vi "OSC UDP Receiver.vi"() -> ()   [LabVIEW 2013]
doc: "This example VI shows how to read Open Sound Control (OSC) messages from UDP and dispatch them by their OSC address patterns. This VI is intended to be run with the OSC UDP Sender example VI."
uses:
  <vilib>/NIOSC/Argument to Float32 Data.vi
  <vilib>/NIOSC/Argument to Boolean Data.vi
  <vilib>/NIOSC/Argument to String Data.vi
  <vilib>/NIOSC/Argument to Double Data.vi
  <vilib>/NIOSC/Generate Error.vi
  <vilib>/NIOSC/Check for Valid String Data.vi
  <vilib>/NIOSC/NI_OSC.lvlib
panel:
  out "float32 data 3":sgl format="%.3f"
  out "float32 data 2":sgl format="%.3f"
  out "Stop Button":sgl
  out "float32 data":sgl format="%.3f"
  out "/group4/data":T1
  out "Zaxis":sgl(slide) scale=-1.0..1.0
  in  "stop":bool
  in  "Local Port":u16=9000
  # "Instructions:\n1. Open the sender VI (OSC UDP Sender.vi).\n2. Make sure the Remote Port in the sender VI and the Local Port in this VI are the same.\n3. Run both VIs.\n4. Change the values of the controls on the sender VI.  The indicators in this VI with the corresponding method addresses should update."
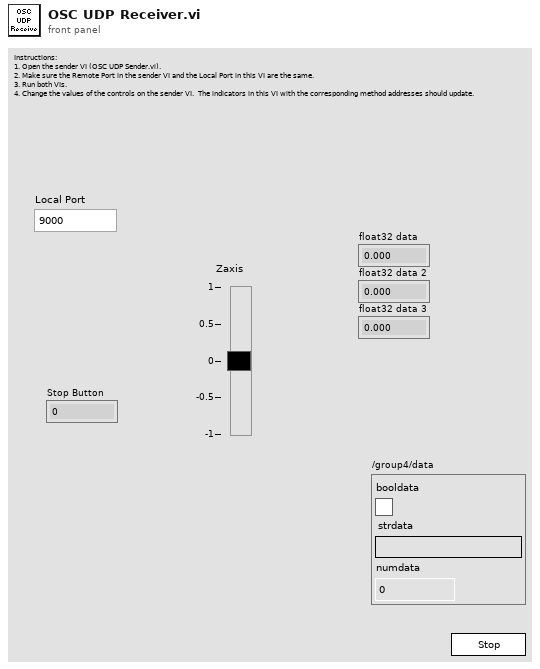
[diagram p1: front panel]
types:
  T1 = cluster{"booldata":bool, "strdata":string, "numdata":dbl}
  T2 = typedef "NI_OSC.lvlib/Address Space Node.ctl" = cluster{"parent index":i32, "child indexes":i32[], "address part":string, "method":bool, "data":variant}
  T3 = typedef "NI_OSC.lvlib/Method Dispatching Info.ctl" = cluster{"method address":string, "message":string, "message timetag":u64, "data":variant}
  T4 = typedef "NI_OSC.lvlib/Argument.ctl" = cluster{"argument":string, "type tag":string}
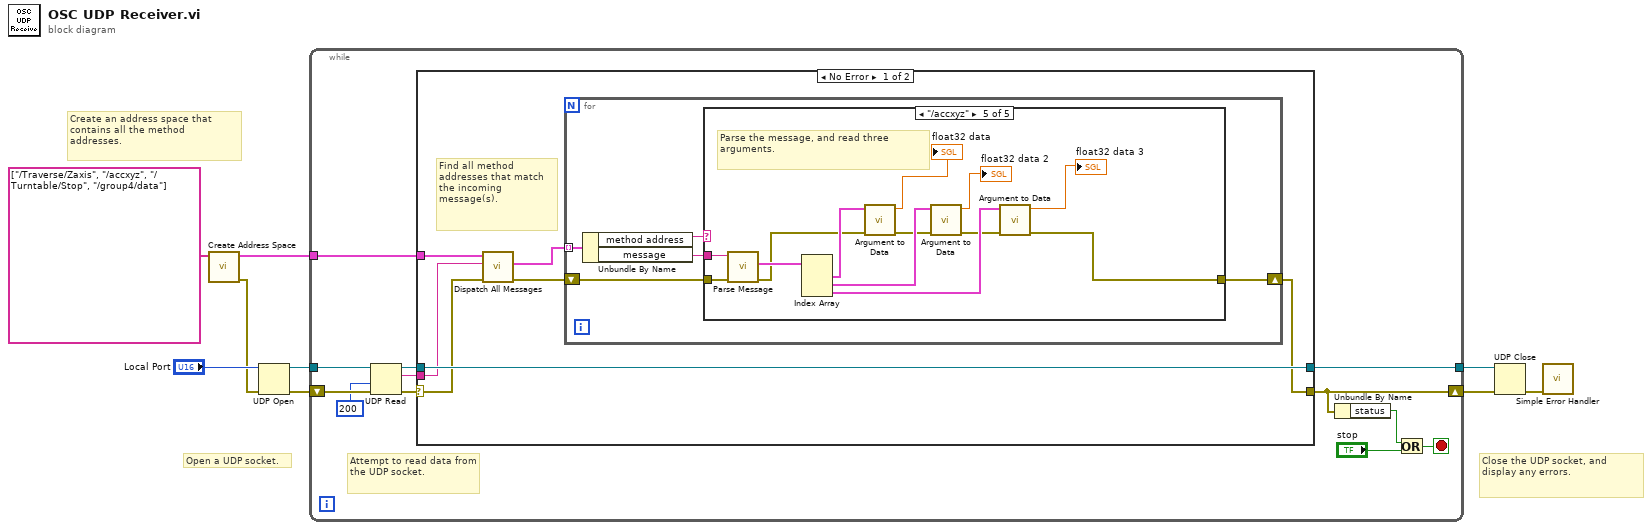
[diagram p0: block diagram]
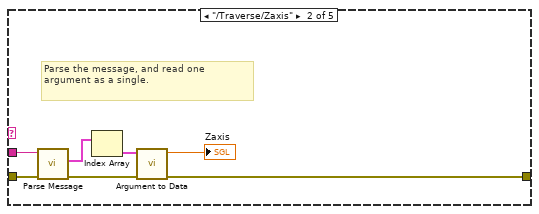
[diagram p3: hidden frame]
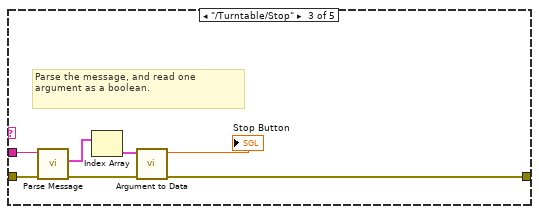
[diagram p4: hidden frame]
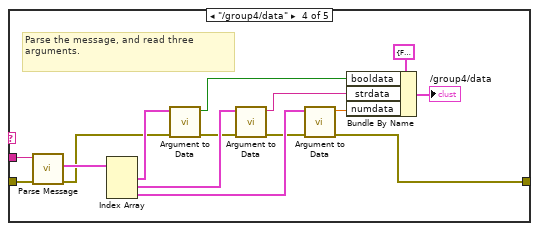
[diagram p5: hidden frame]
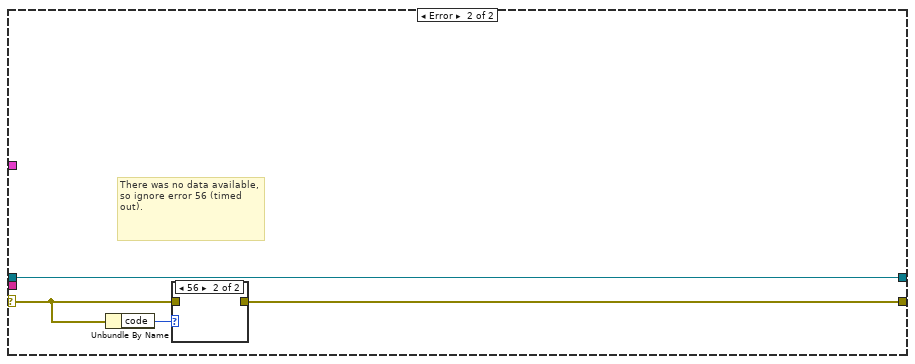
[diagram p6: hidden frame]
diagram:
  # "Close the UDP socket, and display any errors."
  # "Open a UDP socket."
  # "Create an address space that contains all the method addresses."
  n1 = call <vilib>:"Create Address Space.vi"("method addresses"=string[] ["/Traverse/Zaxis", "/accxyz", "/Turntable/Stop", "/group4/data"]) -> ("error out"=w1:errorcluster, "address space out"=w2:T2[])  [unwired: 9 in]
  n2 = UDP Open(8:w1, 11:"Local Port") -> (port=w8:refnum<k16>, 0:w7:errorcluster)  [unwired: 3 in, 1 out]
  n3 = while {
    tunnel: w8 -> [w19]
    shift-right: [w13] -> w5
    shift-left: w7 -> [w18]
    tunnel: [w14] -> w6
    tunnel: w2 -> [w11]
    stop <- w20 stop-if-true
    # "Attempt to read data from the UDP socket."
    n4 = UDP Read(connection ID=w19, timeout ms (25000)=200, 8:w18) -> (data out=w12:string, error out=w16:errorcluster, 3:w15:refnum<k16>)  [unwired: 1 in, 2 out]
    n5 = case shown="No Error" w16 {
      selector: w16 -> [w25 w79]
      tunnel: w15 -> [w28 w77]
      tunnel: [w28 w77] -> w14
      tunnel: [w22 w78] -> w13
      tunnel: w12 -> [w27 _]
      tunnel: w11 -> [w26 _]
      frame No Error {
        # "Find all method addresses that match the incoming message(s)."
        n6 = call <vilib>:"Dispatch All Messages.vi"("error in"=w25, "packet"=w27, "address space in"=w26) -> ("error out"=w23:errorcluster, "method dispatching info"=w24:T3[])  [unwired: 6 in, 1 out]
        n7 = for {
          tunnel: w24 -> [w33] mode=indexing
          shift-right: [w31] -> w22
          shift-left: w23 -> [w32]
          n8 = Unbundle By Name(w33) -> ("method address"=w30:string, "message"=w29:string)
          n9 = case shown="\"/accxyz\"" w30 {
            tunnel: w32 -> [w34 w41 w48 w63 w76]
            tunnel: [w34 w37 w44 w50 w67] -> w31
            tunnel: w29 -> [_ w36 w43 w60 w73]
            frame Default {
            }
            frame "/Traverse/Zaxis" {
              # "Parse the message, and read one argument as a single."
              n10 = call <vilib>:"Parse Message.vi"("error in"=w41, "message"=w36) -> ("error out"=w38:errorcluster, "arguments"=w40:T4[])  [unwired: 7 in, 1 out]
              n11 = Index Array(array=w40) -> (element=w39:T4)  [unwired: 1 in]
              n12 = call-poly <vilib>:"Argument to Data.vi"("error in"=w38, "float32 argument"=w39) -> ("error out"=w37:errorcluster, "float32 data"=→"Zaxis":sgl)  [unwired: 8 in]
            }
            frame "/Turntable/Stop" {
              # "Parse the message, and read one argument as a boolean."
              n13 = call <vilib>:"Parse Message.vi"("error in"=w48, "message"=w43) -> ("error out"=w45:errorcluster, "arguments"=w47:T4[])  [unwired: 7 in, 1 out]
              n14 = Index Array(array=w47) -> (element=w46:T4)  [unwired: 1 in]
              n15 = call-poly <vilib>:"Argument to Data.vi"("error in"=w45, "float32 argument"=w46) -> ("error out"=w44:errorcluster, "float32 data"=→"Stop Button":sgl)  [unwired: 8 in]
            }
            frame "/group4/data" {
              # "Parse the message, and read three arguments."
              n16 = call <vilib>:"Parse Message.vi"("error in"=w63, "message"=w60) -> ("error out"=w49:errorcluster, "arguments"=w62:T4[])  [unwired: 7 in, 1 out]
              n17 = Index Array(array=w62) -> (element #1=w61:T4, element #2=w56:T4, element #3=w54:T4)  [unwired: 3 in]
              n18 = call-poly <vilib>:"Argument to Data.vi"("error in"=w49, "boolean argument"=w61) -> ("error out"=w51:errorcluster, "boolean data"=w57:bool)  [unwired: 8 in]
              n19 = call-poly <vilib>:"Argument to Data.vi"("error in"=w51, "string argument"=w56) -> ("error out"=w52:errorcluster, "string data"=w55:string)  [unwired: 8 in]
              n20 = call-poly <vilib>:"Argument to Data.vi"("error in"=w52, "double argument"=w54) -> ("error out"=w50:errorcluster, "double data"=w53:dbl)  [unwired: 8 in]
              n21 = Bundle By Name(cluster=T1 {"booldata"=FALSE, "strdata"="", "numdata"=0.0} ("/group4/data"), "booldata"=w57, "strdata"=w55, "numdata"=w53) -> (→"/group4/data":T1)
            }
            frame "/accxyz" {
              # "Parse the message, and read three arguments."
              n22 = call <vilib>:"Parse Message.vi"("error in"=w76, "message"=w73) -> ("error out"=w66:errorcluster, "arguments"=w75:T4[])  [unwired: 7 in, 1 out]
              n23 = Index Array(array=w75) -> (element #1=w74:T4, element #2=w71:T4, element #3=w70:T4)  [unwired: 3 in]
              n24 = call-poly <vilib>:"Argument to Data.vi"("error in"=w66, "float32 argument"=w74) -> ("error out"=w68:errorcluster, "float32 data"=→"float32 data":sgl)  [unwired: 8 in]
              n25 = call-poly <vilib>:"Argument to Data.vi"("error in"=w68, "float32 argument"=w71) -> ("error out"=w69:errorcluster, "float32 data"=→"float32 data 2":sgl)  [unwired: 8 in]
              n26 = call-poly <vilib>:"Argument to Data.vi"("error in"=w69, "float32 argument"=w70) -> ("error out"=w67:errorcluster, "float32 data"=→"float32 data 3":sgl)  [unwired: 8 in]
            }
          }
        }
      }
      frame Error {
        # "There was no data available, so ignore error 56 (timed out)."
        n27 = Unbundle By Name(w79) -> ("code"=w80:i32)
        n28 = case shown="56" w80 {
          tunnel: w79 -> [w81 _]
          tunnel: [w81 _] -> w78
          frame Default {
          }
          frame 56 {
          }
        }
      }
    }
    n29 = Unbundle By Name(w13) -> ("status"=w21:bool)
    n30 = Or(x=w21, y="stop") -> (x .or. y?=w20:bool)
  }
  n31 = UDP Close(connection ID=w6, 8:w5) -> (error out=w4:errorcluster)  [unwired: 1 out]
  n32 = call <vilib>:"Simple Error Handler.vi"("error in (no error)"=w4) -> ()  [unwired: 4 in, 5 out]
